vi "Calc_Normalize Value.vi"(0 "Value":dbl, 7 "Max":dbl, 9 "Min":dbl) -> (14 "Normalized Value":dbl)   [LabVIEW 2017]
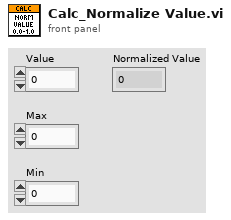
[diagram p1: front panel]
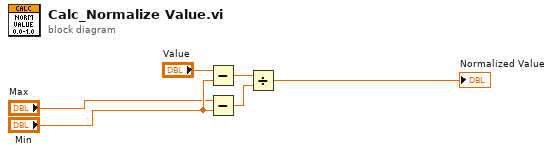
[diagram p0: block diagram]
diagram:
  n1 = Subtract(x="Value", y="Min") -> (x-y=w2:dbl)
  n2 = Subtract(x="Max", y="Min") -> (x-y=w3:dbl)
  n3 = Divide(x=w2, y=w3) -> (x/y=→"Normalized Value":dbl)
